vi "Test.vi"() -> ()   [LabVIEW 2020, in "AK-Schnittstelle.lvlib"]
uses:
  AK-Schnittstelle.lvlib
panel:
  out "Dezimalziffer?":bool
  out "Zahl 2":dbl format="%#.6g"
  out "Zahl":i32
  # "Fertiger String wie es bei uns Angezeigt wird"
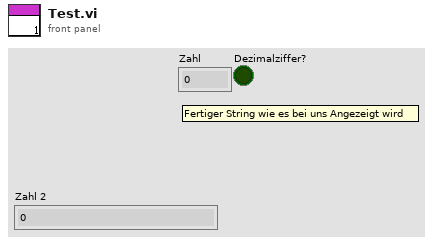
[diagram p1: front panel]
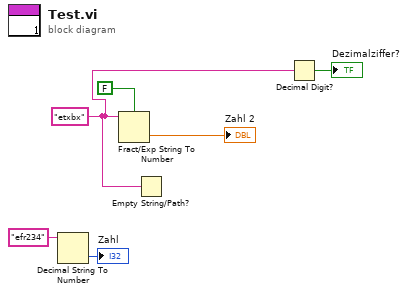
[diagram p0: block diagram]
diagram:
  w2 = "etxbx" ("String")
  n1 = Decimal String To Number(string="efr234" ("String")) -> (number=→"Zahl":i32)  [unwired: 2 in, 1 out]
  n2 = Fract/Exp String To Number(use system decimal point (T)=FALSE ("Systemdezimalzeichen verwenden (T)"), string=w2) -> (number=→"Zahl 2":dbl)  [unwired: 2 in, 1 out]
  n3 = Empty String/Path?(string/path=w2) -> ()  [unwired: 1 out]
  n4 = Decimal Digit?(1:w2) -> (0:→"Dezimalziffer?":bool)
